vi "array to chconfig.vi"(9 "output array":string[][](array[string])=array264x16[4224 elements]) -> (1 "configtable":T1 {"CHS"."display" format="%b"})   [LabVIEW 2011]
uses:
  gain.ctl
  contable.ctl
  CHS.ctl
  singlechtype.ctl
panel:
  in  "Gain":T4
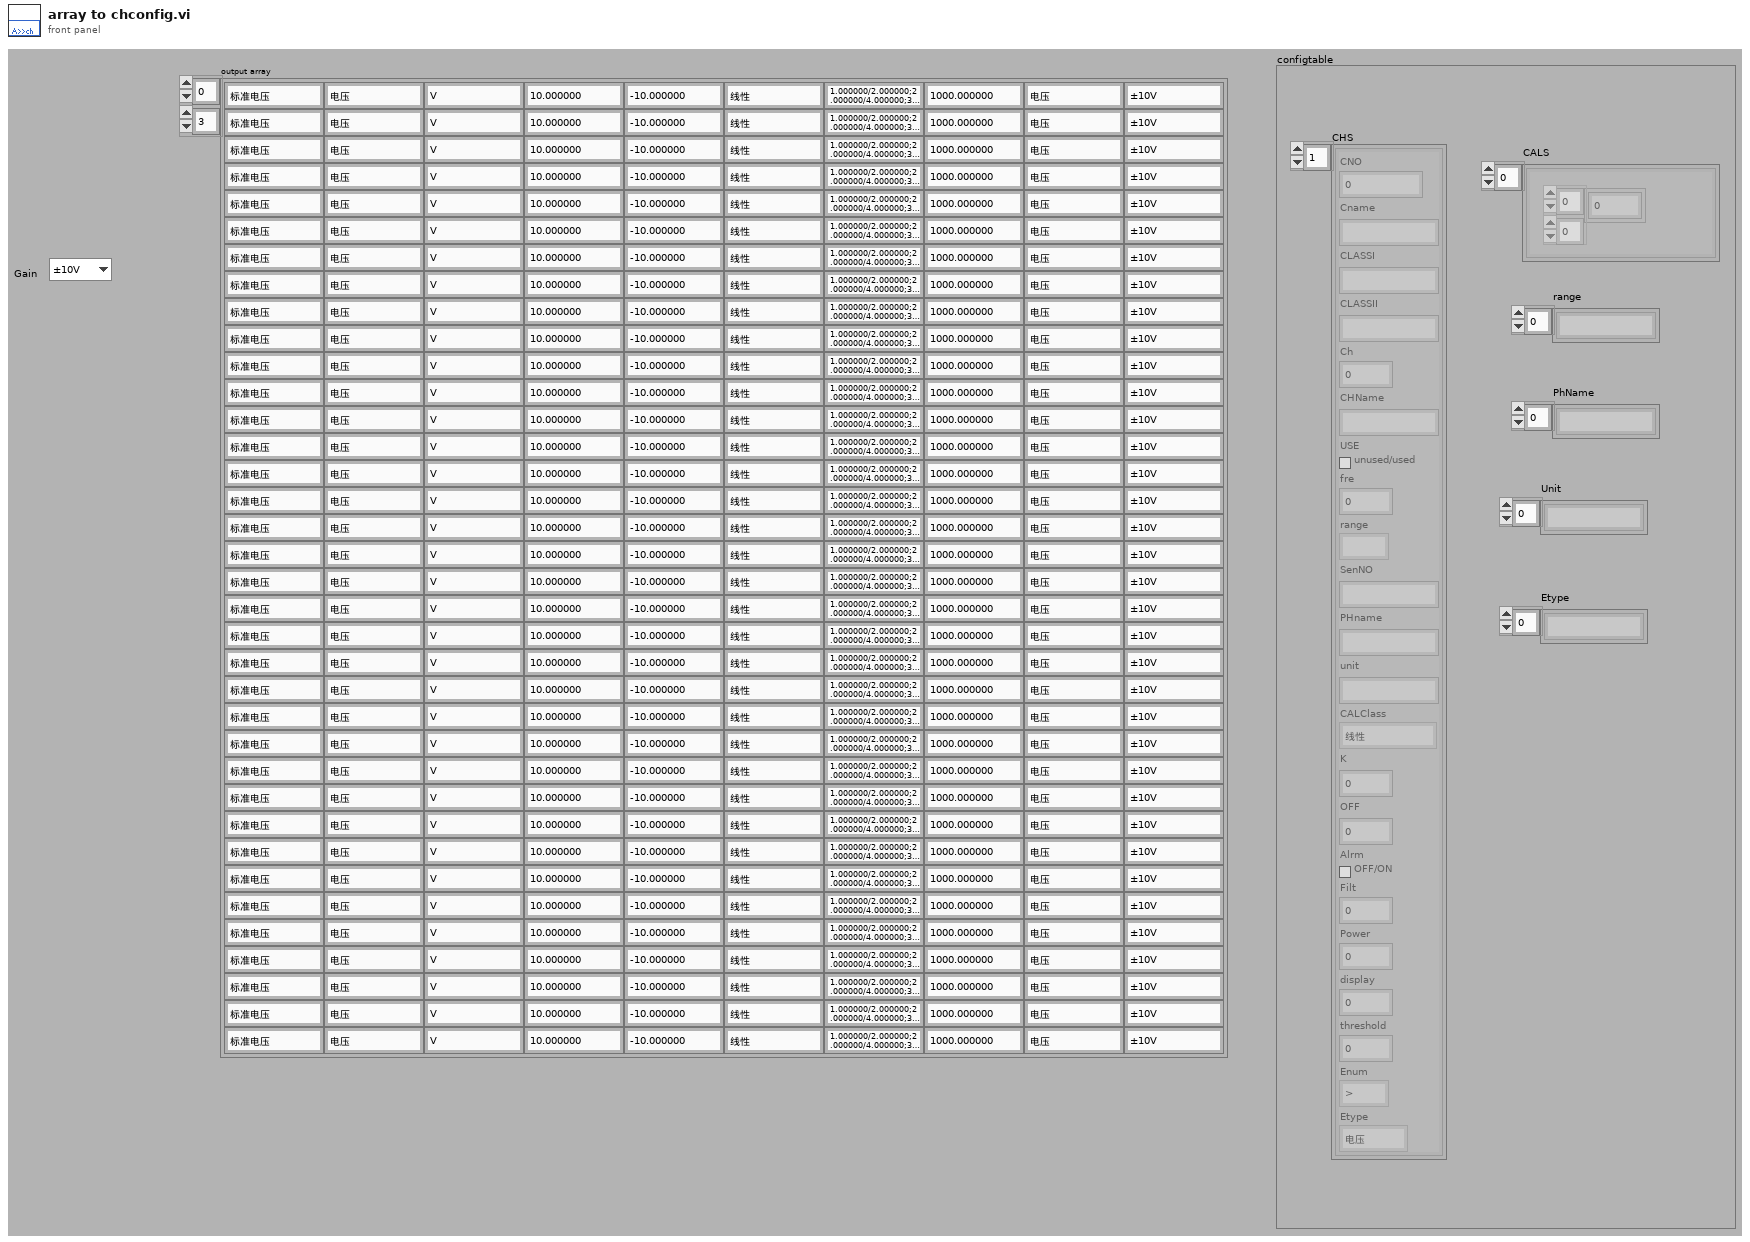
[diagram p1: front panel]
types:
  T1 = typedef "contable.ctl" = cluster{"CHS":T2, "CALS":cluster{"Array":dbl[][]}[], "range":string[], "PhName":string[], "Unit":string[], "Etype":string[]}
  T2 = typedef "CHS.ctl" = T3[]
  T3 = typedef "singlechtype.ctl" = cluster{"CNO":u8, "Cname":string, "CLASSI":string, "CLASSII":string, "Ch":u8, "CHName":string, "USE":bool, "fre":dbl, "range":enum16{""}, "SenNO":string, "PHname":string, "unit":string, "CALClass":enum8{"线性", "查表", "公式"}, "K":dbl, "OFF":dbl, "Alrm":bool, "Filt":dbl, "Power":u8, "display":u8, "threshold ":dbl, "Enum":enum16{">", ">=", "<", "<=", "<>(在范围内）", "><（在范围外）"}, "Etype":enum16{"电压", "电流", "电阻", "热电偶K", "热电偶T"}}
  T4 = typedef "gain.ctl" = enum16{"±10V", "±5V", "±2.5V", "±1V", "±500mV", "±100mV", "10V", "5V", "2.5V", "1V", "500mV", "100mV"}
  T5 = typedef "chdatatype.ctl" = cluster{"dataname":string, "datavalue":T6, "Find":bool}
  T6 = typedef "config table enum.ctl" = enum16{"CNO.", "CName", "CLASSI", "CLASSII", "ch", "Chname", "USE", "fre", "range", "senNO", "PHname", "unit", "CALclass", "K", "OFF", "Alrm", "filt", "Power", "display", "threshold", "compare", "Etype"}
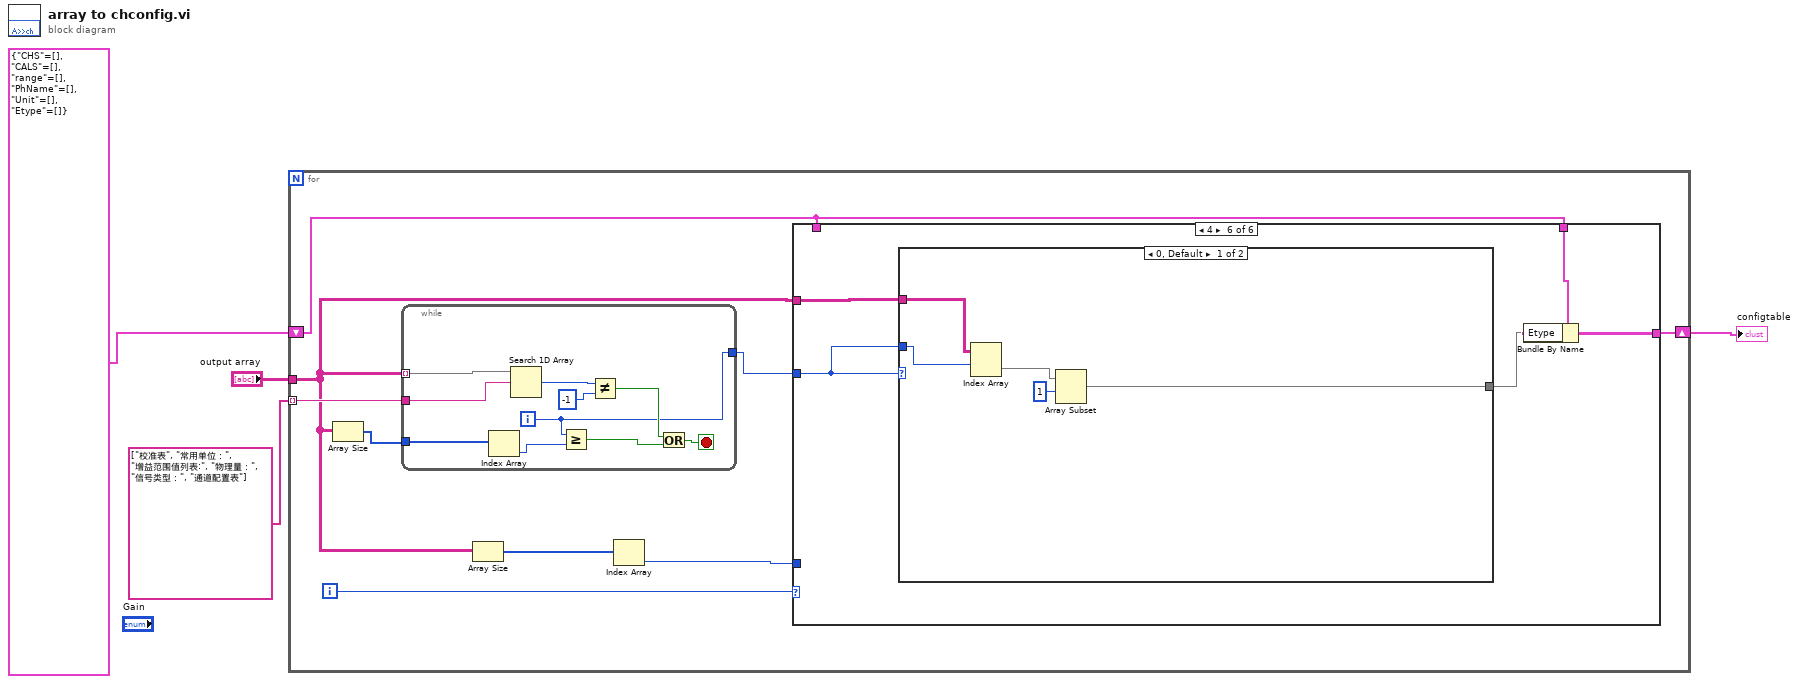
[diagram p0: block diagram]
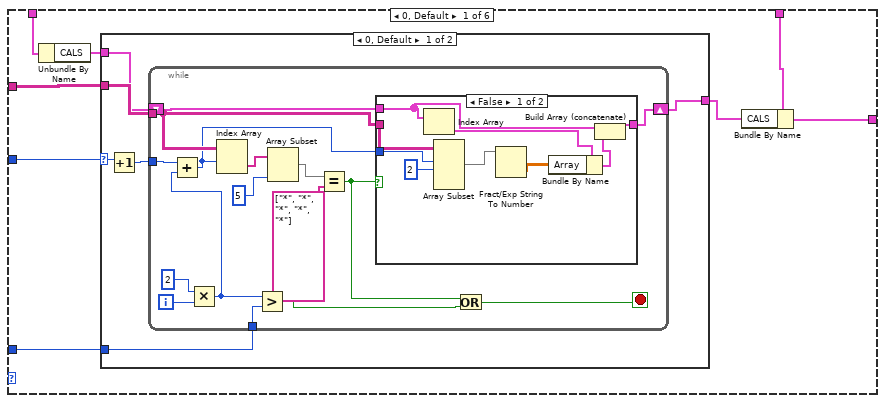
[diagram p2: hidden frame]
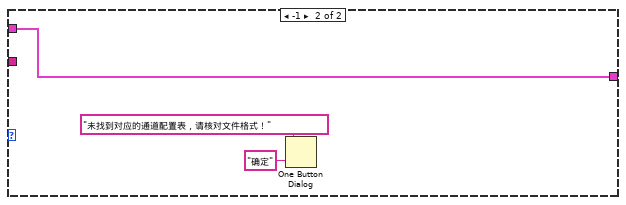
[diagram p4: hidden frame]
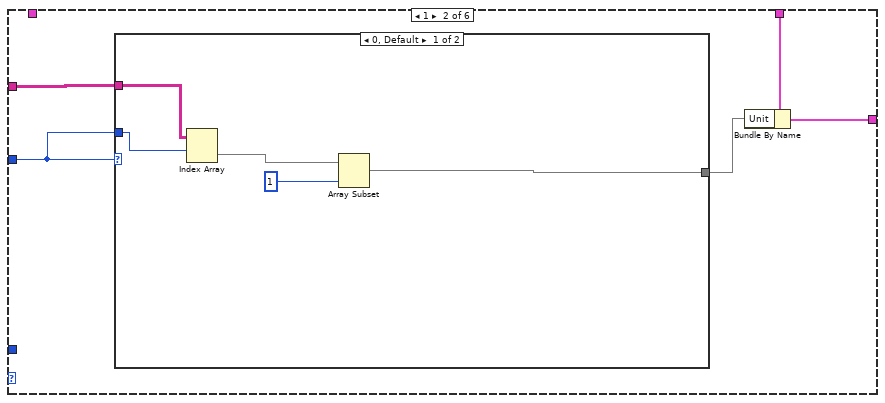
[diagram p5: hidden frame]
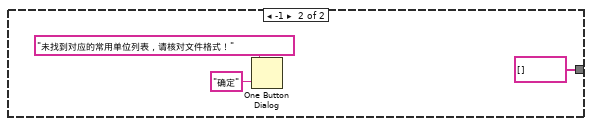
[diagram p6: hidden frame]
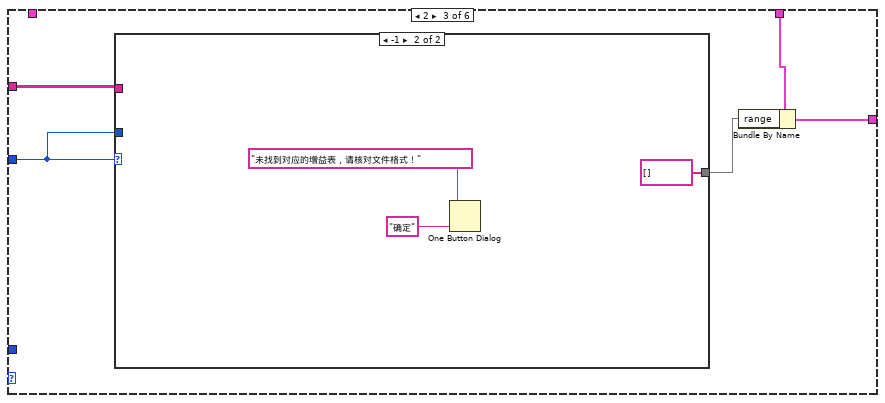
[diagram p7: hidden frame]
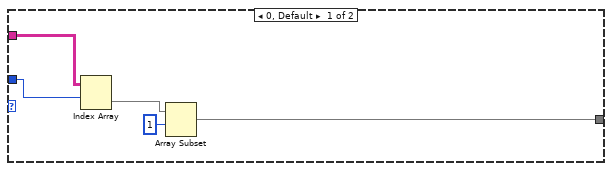
[diagram p8: hidden frame]
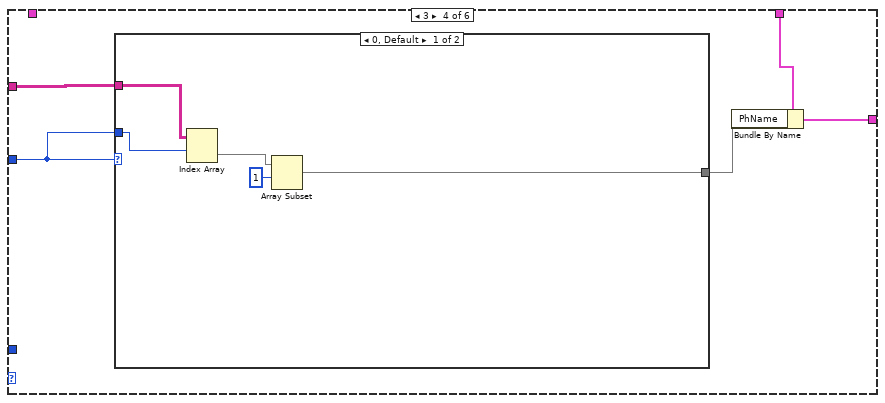
[diagram p9: hidden frame]
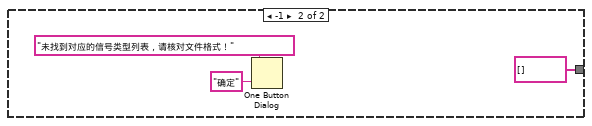
[diagram p10: hidden frame]
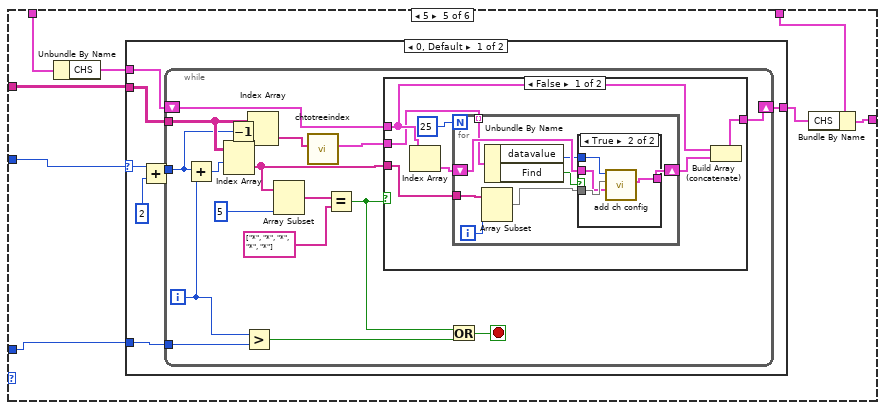
[diagram p11: hidden frame]
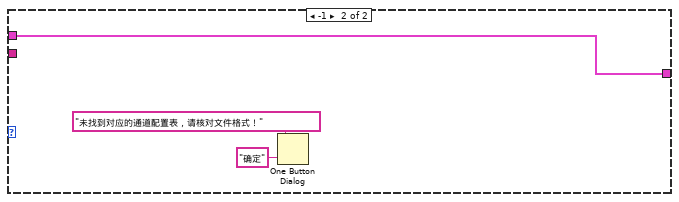
[diagram p14: hidden frame]
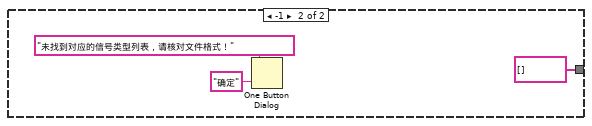
[diagram p15: hidden frame]
diagram:
  n1 = for {
    tunnel: "output array" -> [w7]
    tunnel: string[] ["校准表", "常用单位：", "增益范围值列表:", "物理量：", "信号类型：", "通道配置表"] -> [w11] mode=indexing
    shift-right: [w8] -> w1
    shift-left: T1 {"CHS"=[], "CALS"=[], "range"=[], "PhName"=[], "Unit"=[], "Etype"=[]} ("configtable") -> [w9]
    i -> [w10]
    n2 = Array Size(array=w7) -> (size(s)=w12:i32[])
    n3 = while {
      tunnel: w7 -> [w174] mode=indexing
      tunnel: w12 -> [w173]
      tunnel: [w165] -> w13
      tunnel: w11 -> [w166]
      i -> [w165]
      stop <- w170 stop-if-true
      n4 = Index Array(array=w173) -> (element=w172:i32)  [unwired: 1 in]
      n5 = Search 1D Array(1D array=w174, element=w166) -> (index of element=w167:i32)  [unwired: 1 in]
      n6 = Greater Or Equal?(x=w165, y=w172) -> (x >= y?=w168:bool)
      n7 = Not Equal?(x=w167, y=-1) -> (x != y?=w169:bool)
      n8 = Or(x=w169, y=w168) -> (x .or. y?=w170:bool)
    }
    n9 = Array Size(array=w7) -> (size(s)=w6:i32[])
    n10 = Index Array(array=w6) -> (element=w5:i32)  [unwired: 1 in]
    n11 = case shown="4" w10 {
      tunnel: w13 -> [w21 w61 w74 w87 w103 w156]
      tunnel: w7 -> [w20 w60 w73 w86 w102 w155]
      tunnel: [w19 w59 w72 w85 w101 w154] -> w8
      tunnel: w9 -> [w18 w58 w71 w84 w100 w153]
      tunnel: w9 -> [w17 _ _ _ w98 _]
      tunnel: w5 -> [w14 _ _ _ w96 _]
      frame 0, Default {
        n12 = Unbundle By Name(w17) -> ("CALS"=w16:cluster{"Array":dbl[][]}[])
        n13 = case shown="0, Default" w21 {
          selector: w21 -> [w23 _]
          tunnel: w20 -> [w27 _]
          tunnel: w16 -> [w25 w54]
          tunnel: [w24 w54] -> w15
          tunnel: w14 -> [w22 _]
          frame 0, Default {
            n14 = Increment(x=w23) -> (x+1=w26:i32)
            n15 = while {
              tunnel: w27 -> [w34]
              tunnel: w26 -> [w39]
              shift-right: [w35] -> w24
              shift-left: w25 -> [w36]
              tunnel: w22 -> [w31]
              i -> [w38]
              stop <- w28 stop-if-true
              n16 = Multiply(x=2, y=w38) -> (x*y=w32:i32)
              n17 = Add(x=w39, y=w32) -> (x+y=w33:i32)
              n18 = Index Array(array=w34, index (row)=w33) -> (element=w42:string[])  [unwired: 1 in]
              n19 = Greater?(x=w32, y=w31) -> (0:w29:bool)
              n20 = Array Subset(array=w42, length=5) -> (w40:string[])  [unwired: 1 in]
              n21 = Equal?(x=w40, y=string[] ["*", "*", "*", "*", "*"]) -> (x = y?=w30:bool)
              n22 = case shown="False" w30 {
                tunnel: w36 -> [w47 w53]
                tunnel: [w46 w53] -> w35
                tunnel: w34 -> [w52 _]
                tunnel: w33 -> [w51 _]
                frame False {
                  n23 = Index Array(array=w47) -> (element=w45:cluster{"Array":dbl[][]})  [unwired: 1 in]
                  n24 = Array Subset(array=w52, index (row)=w51, length (row)=2 ("length")) -> (w49:string[][])  [unwired: 2 in]
                  n25 = Fract/Exp String To Number(string=w49) -> (number=w48:dbl[][])  [unwired: 3 in, 1 out]
                  n26 = Bundle By Name(cluster=w45, "Array"=w48) -> (w44:cluster{"Array":dbl[][]})
                  n27 = Build Array (concatenate)(w47, w44) -> (w46:cluster{"Array":dbl[][]}[])
                }
                frame True {
                }
              }
              n28 = Or(x=w30, y=w29) -> (x .or. y?=w28:bool)
            }
          }
          frame -1 {
            n29 = One Button Dialog(message="未找到对应的通道配置表，请核对文件格式！", button name ("OK")="确定") -> ()  [unwired: 1 out]
          }
        }
        n30 = Bundle By Name(cluster=w18, "CALS"=w15) -> (w19:T1)
      }
      frame 1 {
        n31 = case shown="0, Default" w61 {
          tunnel: w60 -> [w66 _]
          tunnel: w61 -> [w65 _]
          tunnel: [w62 string[] []] -> w57
          frame 0, Default {
            n32 = Index Array(array=w66, index (row)=w65) -> (element=w64:string[])  [unwired: 1 in]
            n33 = Array Subset(array=w64, index=1) -> (w62:string[])  [unwired: 1 in]
          }
          frame -1 {
            n34 = One Button Dialog(message="未找到对应的常用单位列表，请核对文件格式！", button name ("OK")="确定") -> ()  [unwired: 1 out]
          }
        }
        n35 = Bundle By Name(cluster=w58, "Unit"=w57) -> (w59:T1)
      }
      frame 2 {
        n36 = case shown="-1" w74 {
          tunnel: w73 -> [w79 _]
          tunnel: w74 -> [w78 _]
          tunnel: [w75 string[] []] -> w70
          frame 0, Default {
            n37 = Index Array(array=w79, index (row)=w78) -> (element=w77:string[])  [unwired: 1 in]
            n38 = Array Subset(array=w77, index=1) -> (w75:string[])  [unwired: 1 in]
          }
          frame -1 {
            n39 = One Button Dialog(message="未找到对应的增益表，请核对文件格式！", button name ("OK")="确定") -> ()  [unwired: 1 out]
          }
        }
        n40 = Bundle By Name(cluster=w71, "range"=w70) -> (w72:T1)
      }
      frame 3 {
        n41 = case shown="0, Default" w87 {
          tunnel: w86 -> [w92 _]
          tunnel: w87 -> [w91 _]
          tunnel: [w88 string[] []] -> w83
          frame 0, Default {
            n42 = Index Array(array=w92, index (row)=w91) -> (element=w90:string[])  [unwired: 1 in]
            n43 = Array Subset(array=w90, index=1) -> (w88:string[])  [unwired: 1 in]
          }
          frame -1 {
            n44 = One Button Dialog(message="未找到对应的信号类型列表，请核对文件格式！", button name ("OK")="确定") -> ()  [unwired: 1 out]
          }
        }
        n45 = Bundle By Name(cluster=w84, "PhName"=w83) -> (w85:T1)
      }
      frame 5 {
        n46 = Unbundle By Name(w98) -> ("CHS"=w97:T2)
        n47 = case shown="0, Default" w103 {
          selector: w103 -> [w105 _]
          tunnel: w102 -> [w110 _]
          tunnel: w97 -> [w109 w149]
          tunnel: [w108 w149] -> w99
          tunnel: w96 -> [w104 _]
          frame 0, Default {
            n48 = Add(x=w105, y=2 ("x")) -> (x+y=w107:i32)
            n49 = while {
              tunnel: w110 -> [w115]
              tunnel: w107 -> [w113]
              shift-right: [w126] -> w108
              shift-left: w109 -> [w127]
              tunnel: w104 -> [w118]
              i -> [w119]
              stop <- w116 stop-if-true
              n50 = Add(x=w113, y=w119) -> (x+y=w122:i32)
              n51 = Index Array(array=w115, index (row)=w122) -> (element=w121:string[])  [unwired: 1 in]
              n52 = Decrement(x=w113) -> (x-1=w114:i32)
              n53 = Greater?(x=w119, y=w118) -> (0:w117:bool)
              n54 = Index Array(array=w115, index (row)=w114) -> (element=w112:string[])  [unwired: 1 in]
              n55 = Array Subset(array=w121, length=5) -> (w123:string[])  [unwired: 1 in]
              n56 = call "chtotreeindex.vi"("name"=w112) -> ("datatypeindex"=w111:T5[])  [unwired: 10 in]
              n57 = Equal?(x=w123, y=string[] ["*", "*", "*", "*", "*"]) -> (x = y?=w120:bool)
              n58 = case shown="False" w120 {
                tunnel: w127 -> [w132 w148]
                tunnel: [w131 w148] -> w126
                tunnel: w121 -> [w134 _]
                tunnel: w111 -> [w128 _]
                frame False {
                  n59 = Index Array(array=w132) -> (element=w133:T3)  [unwired: 1 in]
                  n60 = for {
                    N: 25 -> [_]
                    shift-right: [w139] -> w130
                    shift-left: w133 -> [w138]
                    tunnel: w134 -> [w142]
                    tunnel: w128 -> [w137] mode=indexing
                    i -> [w141]
                    n61 = Array Subset(array=w142, index=w141) -> (w140:string[])  [unwired: 1 in]
                    n62 = Unbundle By Name(w137) -> ("datavalue"=w136:T6, "Find"=w135:bool)
                    n63 = case shown="True" w135 {
                      tunnel: w140 -> [_ w147]
                      tunnel: [w143 w146] -> w139
                      tunnel: w138 -> [w143 w145]
                      tunnel: w136 -> [_ w144]
                      frame False {
                      }
                      frame True {
                        n64 = call "add ch config.vi"("device chanel"=w145, "value"=w147, "Enum"=w144) -> ("device chanel out"=w146:T3)  [unwired: 2 in, 6 out]
                      }
                    }
                  }
                  n65 = Build Array (concatenate)(w132, w130) -> (w131:T2)
                }
                frame True {
                }
              }
              n66 = Or(x=w120, y=w117) -> (x .or. y?=w116:bool)
            }
          }
          frame -1 {
            n67 = One Button Dialog(message="未找到对应的通道配置表，请核对文件格式！", button name ("OK")="确定") -> ()  [unwired: 1 out]
          }
        }
        n68 = Bundle By Name(cluster=w100, "CHS"=w99) -> (w101:T1)
      }
      frame 4 {
        n69 = case shown="0, Default" w156 {
          tunnel: w155 -> [w161 _]
          tunnel: w156 -> [w160 _]
          tunnel: [w157 string[] []] -> w152
          frame 0, Default {
            n70 = Index Array(array=w161, index (row)=w160) -> (element=w159:string[])  [unwired: 1 in]
            n71 = Array Subset(array=w159, index=1) -> (w157:string[])  [unwired: 1 in]
          }
          frame -1 {
            n72 = One Button Dialog(message="未找到对应的信号类型列表，请核对文件格式！", button name ("OK")="确定") -> ()  [unwired: 1 out]
          }
        }
        n73 = Bundle By Name(cluster=w153, "Etype"=w152) -> (w154:T1)
      }
    }
  }
  "configtable" <- w1
